vi "Read standard_name.vi"(8 "error in (no error)":errorcluster, 11 "Pipette in":refnum<class "Pipette.lvclass">) -> (0 "error out":errorcluster, 2 "standard_name":string, 3 "Pipette out":refnum<class "Pipette.lvclass">)   [LabVIEW 2018, in "Pipette.lvclass"]
uses:
  Pipette.lvclass
  Pipette.lvclass/Pipette.ctl
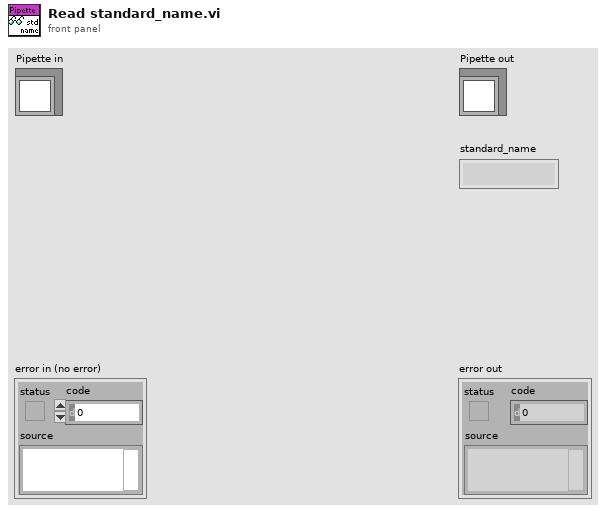
[diagram p1: front panel]
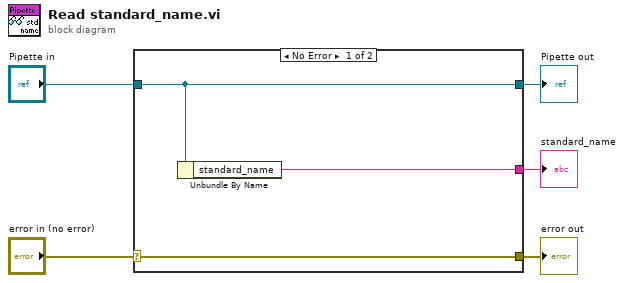
[diagram p0: block diagram]
diagram:
  n1 = case shown="No Error" "error in (no error)" {
    selector: "error in (no error)" -> [w8 w9]
    tunnel: [w8 w9] -> w4
    tunnel: [w7 w10] -> w2
    tunnel: "Pipette in" -> [w7 w10]
    tunnel: [w6 _] -> w1
    frame No Error {
      n2 = Unbundle By Name(w7) -> ("standard_name"=w6:string)
    }
    frame Error {
    }
  }
  "error out" <- w4
  "Pipette out" <- w2
  "standard_name" <- w1
